vi "eMbot Testing Shift Register.vi"() -> ()   [LabVIEW 2011]
uses:
  C:/Users/mouli/Desktop/Desktop Items/Peter/Peter LabView VIs/eMbot testing/eMbot Benchtop Testing/USDQSB.dll
  USDQSB.dll
  Marker Tracking/subVIs/Global Save.vi
  <vilib>/Utility/file.llb/Write To Spreadsheet File (string).vi
panel:
  out "appended path":path
  in  "Trial":dbl=1.0
  out "Execution:State":T1(ring)
  in  "Subject ID":string="A1234"
  in  "Target Time":dbl=60.0
  out "Elspsed Time":dbl
  in  "Save Location":path=path "C:/Users/mouli/Desktop/Desktop Items/Peter/Data/eMbot Data"
  in  "Save":bool
  in  "stop":bool
  out "Matching Output":string[](array[string])
  in  "Plotcount":i32
  in  "Time offset":dbl
  out "Connected":bool
  out "Numeric":i32
  in  "Tab Control":T2(tab)
  in  "error in (no error)":errorcluster
  out "Signed Count":i32
  in  "Resolution 4":i32
  out "error out":errorcluster
  in  "Apply":bool
  in  "Quadrature Mode 4":enum16{"Clock and Direction", "X1", "X2", "X4"}(ring)
  out "Quadrature Mode":string="Clock and Direction"
  out "Counter Mode 4":string="Free Running"
  out "Resolution":i32=1024
  in  "Reset Count":bool caption="Reset"
  in  "Counter Mode":T3(ring)
  out "Index Configuration 4":string="Disabled"
  in  "Index Configuration":T4(ring)
  out "Trigger On Rollover":bool
  in  "OFF 8":bool caption="ON"
  out "Trigger On Rollunder":bool
  out "Trigger On Match":bool
  in  "OFF 9":bool caption="ON"
  in  "OFF 10":bool caption="ON"
  out "Trigger On Index":bool
  in  "OFF 11":bool caption="ON"
  in  "Clear Status":bool caption="Clear"
  out "Unsigned Count":u32
  out "Status (hex)":u32 format="%x"
  out "Rollover":bool
  out "Rollunder":bool
  out "Match":bool
  out "Index":bool
  out "Counter Enabled":bool
  out "Count Increase":bool
  out "Sign Bit Set":bool
  out "Enable Counter":bool=TRUE
  in  "OFF 12":bool=TRUE caption="ON"
  out "Invert Direction":bool=TRUE
  in  "OFF":bool=TRUE caption="ON"
  out "Encoder Count":dbl(knob) scale=0.0..1023.0
  in  "Connect":bool
  out "Connection Status":string
  in  "Port Name i.e. COM3":string="COM4"
  out "ConnectOpened":bool
  out "ConnectOpened 2":bool
  in  "Port Name i.e. COM3 2":string="COM5"
  out "error out 2":errorcluster
  in  "error in (no error) 2":errorcluster
  in  "Reset Count 2":bool caption="Reset"
  out "Encoder Count 2":dbl(knob) scale=0.0..1023.0
  in  "Clear Status 2":bool caption="Clear"
  out "Unsigned Count 2":u32
  out "Sign Bit Set 2":bool
  out "Count Increase 2":bool
  out "Counter Enabled   2":bool
  out "Index 2":bool
  out "Match 2":bool
  out "Rollunder 2":bool
  out "Rollover 2":bool
  out "Status (hex)    2":u32 format="%x"
  out "Invert Direction 2":bool
  out "Enable Counter 2":bool
  out "Trigger On Index 2":bool
  out "Trigger On Match 2":bool
  out "Trigger On Rollunder 2":bool
  out "Trigger On Rollover 2":bool
  out "Index Configuration 2":string="Disabled"
  out "Counter Mode 2":string="Free Running"
  out "Quadrature Mode 2":string="Clock and Direction"
  out "Resolution 2":i32=1024
  in  "Apply 2":bool caption="Apply"
  in  "OFF 2":bool caption="ON"
  in  "OFF 3":bool=TRUE caption="ON"
  in  "OFF 4":bool caption="ON"
  in  "OFF 5":bool caption="ON"
  in  "OFF 6":bool caption="ON"
  in  "OFF 7":bool caption="ON"
  in  "Index Configuration 3":T4(ring)
  in  "Counter Mode 3":T3(ring)
  in  "Quadrature Mode 3":enum16{"Clock and Direction", "X1", "X2", "X4"}(ring)
  out "Signed Count 2":i32
  in  "Resolution 3":i32
  in  "Have Save\nToggle Begin":bool
  in  "Phase":dbl(slide) scale=0.0..180.0
  in  "Amplitude":dbl(slide)=50.0 scale=0.0..180.0
  in  "Frequency":dbl(slide)=5.0 min=0.0 max=10.0 step=0.01 scale=0.0..10.0
  in  "Offset":dbl(slide)=50.0 scale=0.0..180.0
  in  "Slave Arm":bool
  out "Gait 2":cluster{i32, dbl}[](graph)
  out "Plot":cluster{"Gait 2":cluster{i32, dbl}[]}[](graph)
  in  "Begin":bool
  in  "EMG?":bool
  in  "Popup":bool
  in  "Publish":bool
  in  "Notes":string
  # "COM4: Rainbow cord\nCOM5: Purple cord"
  # "Encoder Configuration"
  # "Encoder Status"
  # "Encoder Configuration"
  # "COM 4"
  # "COM 5"
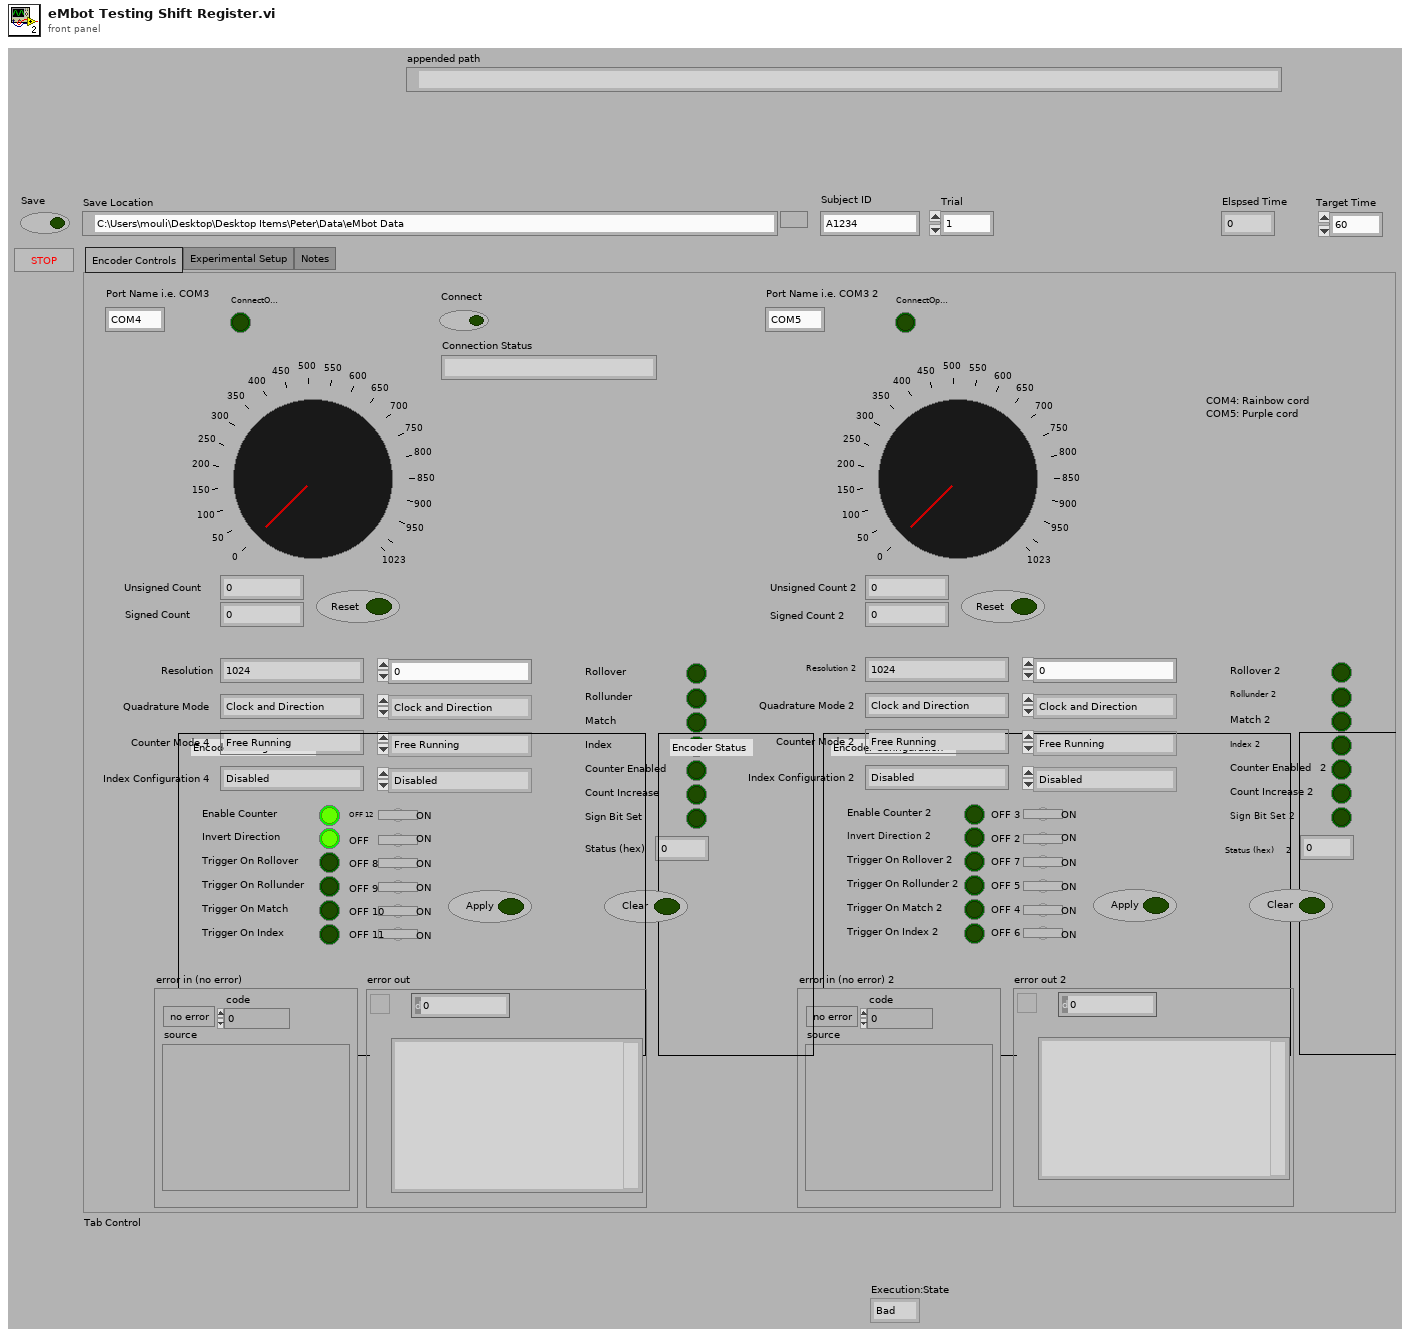
[diagram p1: front panel]
types:
  T1 = enum32{"Bad", "Idle", "Run top level", "Running"}
  T2 = enum32{"Encoder Controls", "Experimental Setup", "Notes"}
  T3 = enum16{"Free Running", "Non-Recycle", "Range Limit", "Modulo-N"}
  T4 = enum16{"Disabled", "Preset Counter", "Reset Counter", "Capture Counter"}
  T5 = enum32{"Invalid", "Standard", "Closed", "Hidden", "Minimized", "Maximized"}
  T6 = typedef "LVDateTimeRec.ctl" = cluster{"fractional second":dbl, "second":i32, "minute":i32, "hour":i32, "day of month":i32, "month":i32, "year":i32, "day of week":i32, "day of year":i32, "DST":i32}
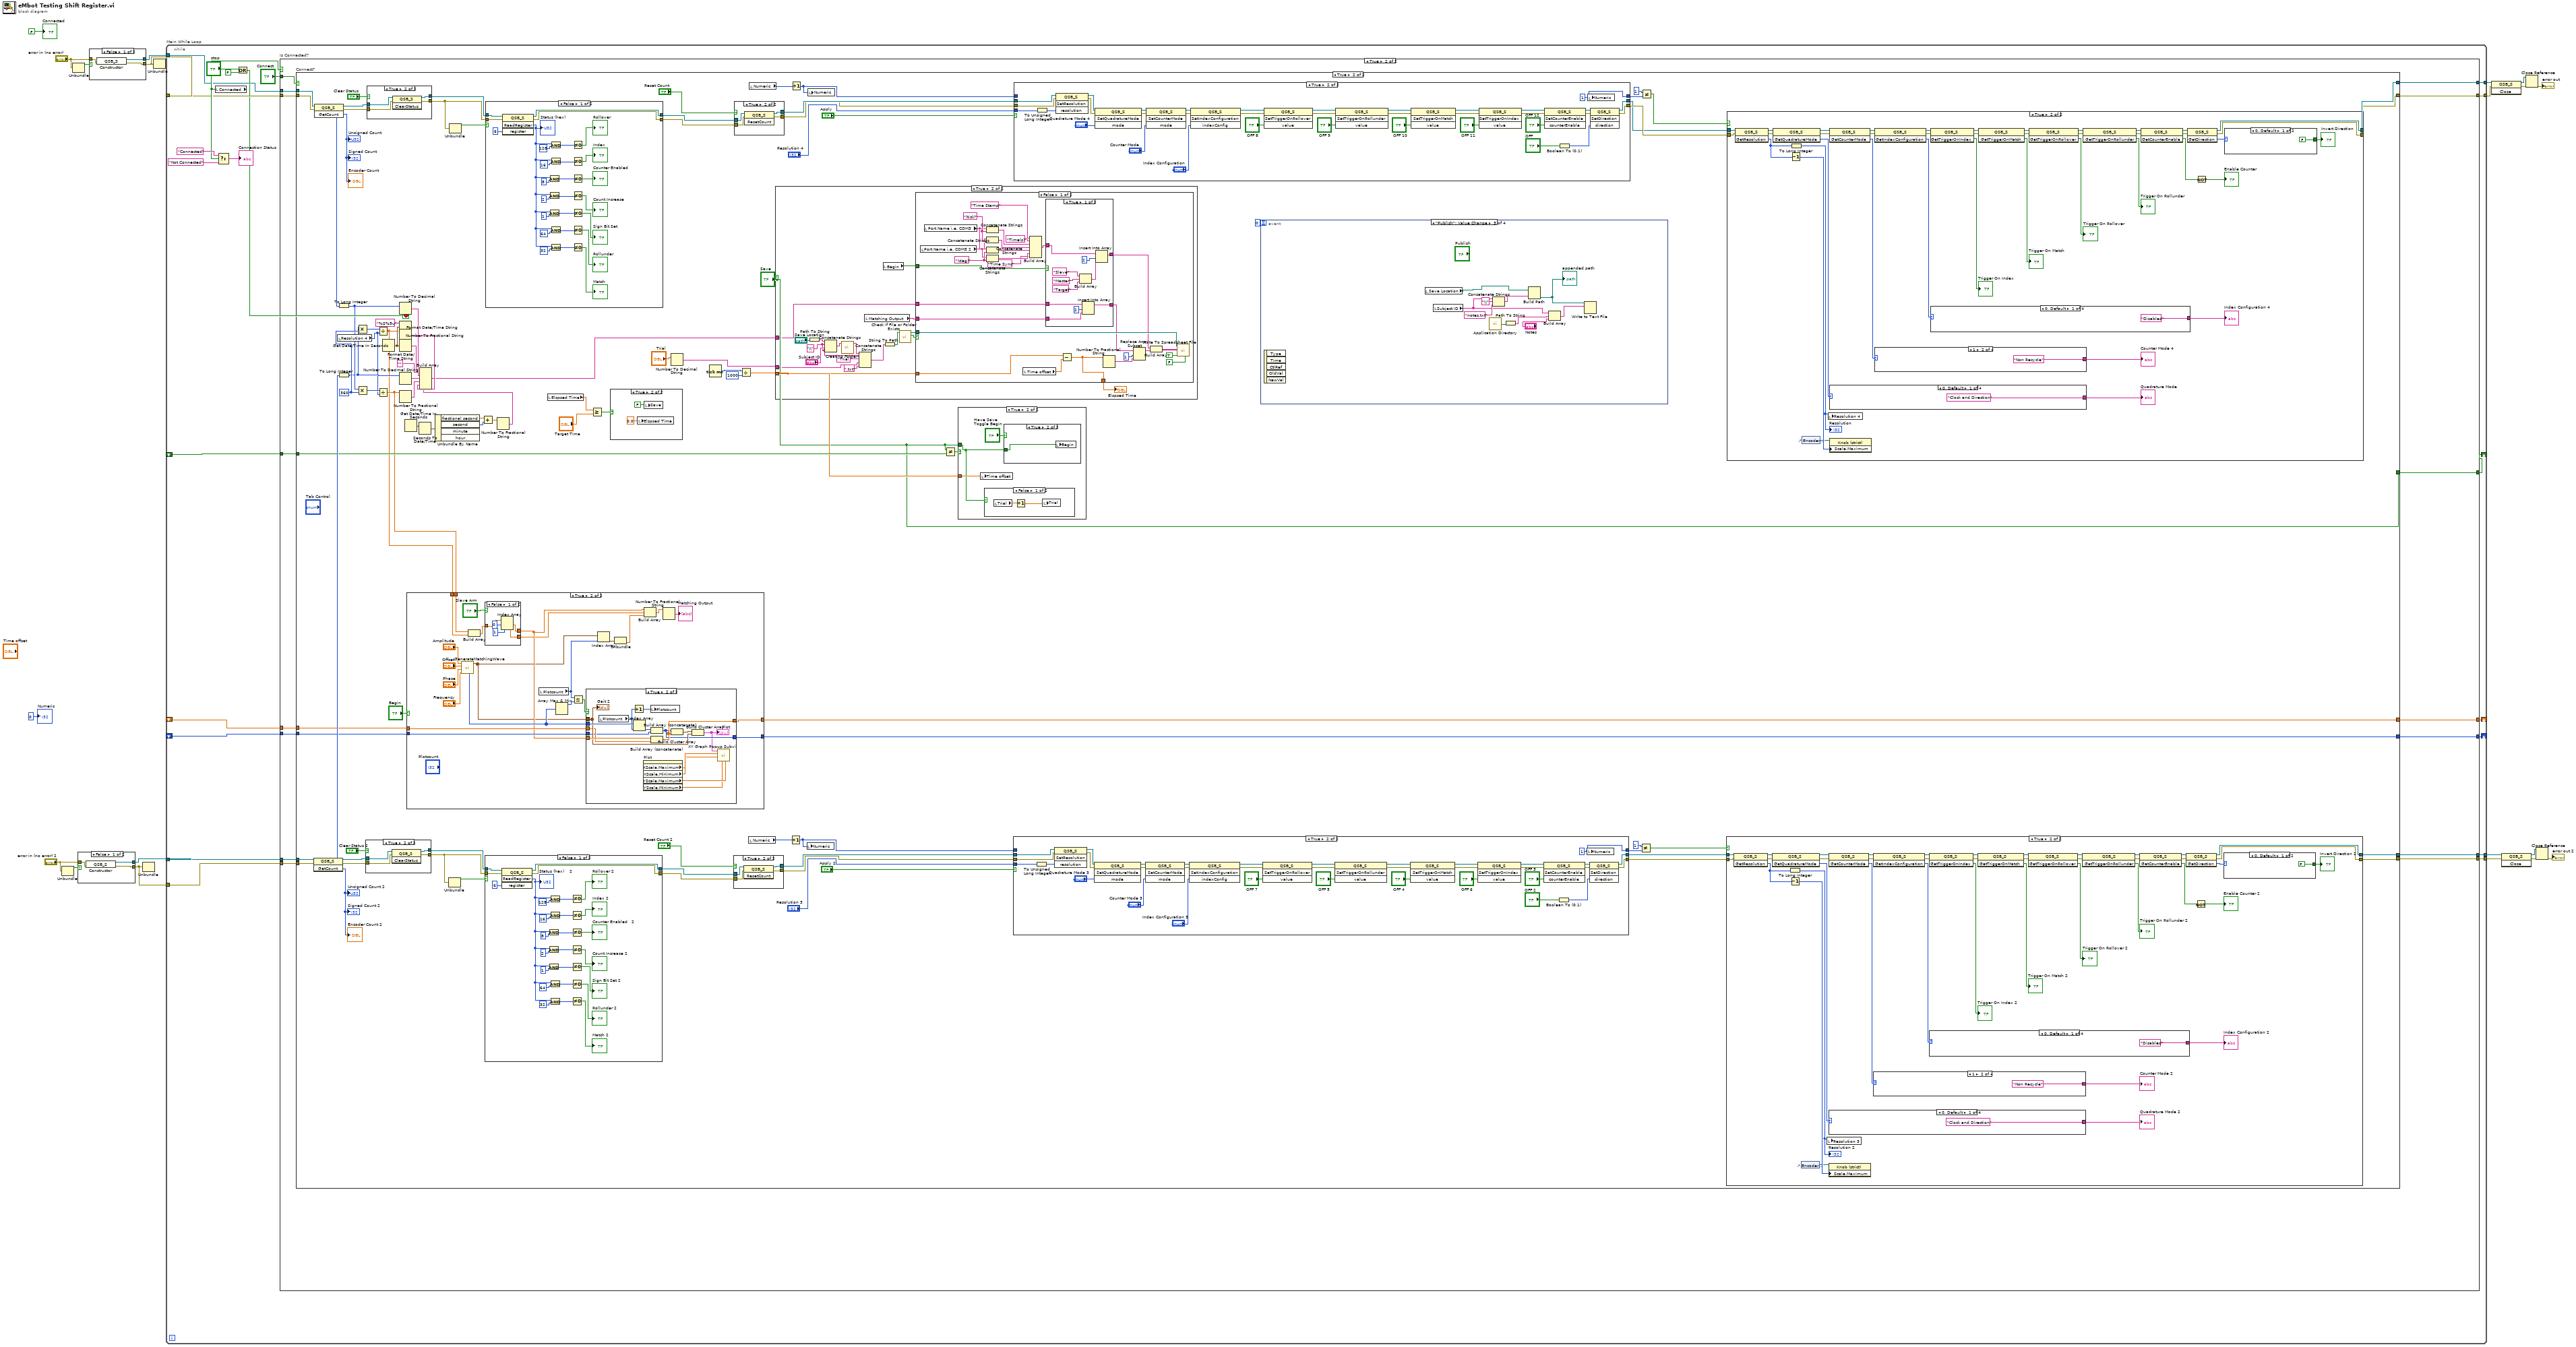
[diagram p0: block diagram]
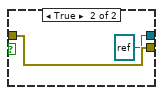
[diagram p2: hidden frame]
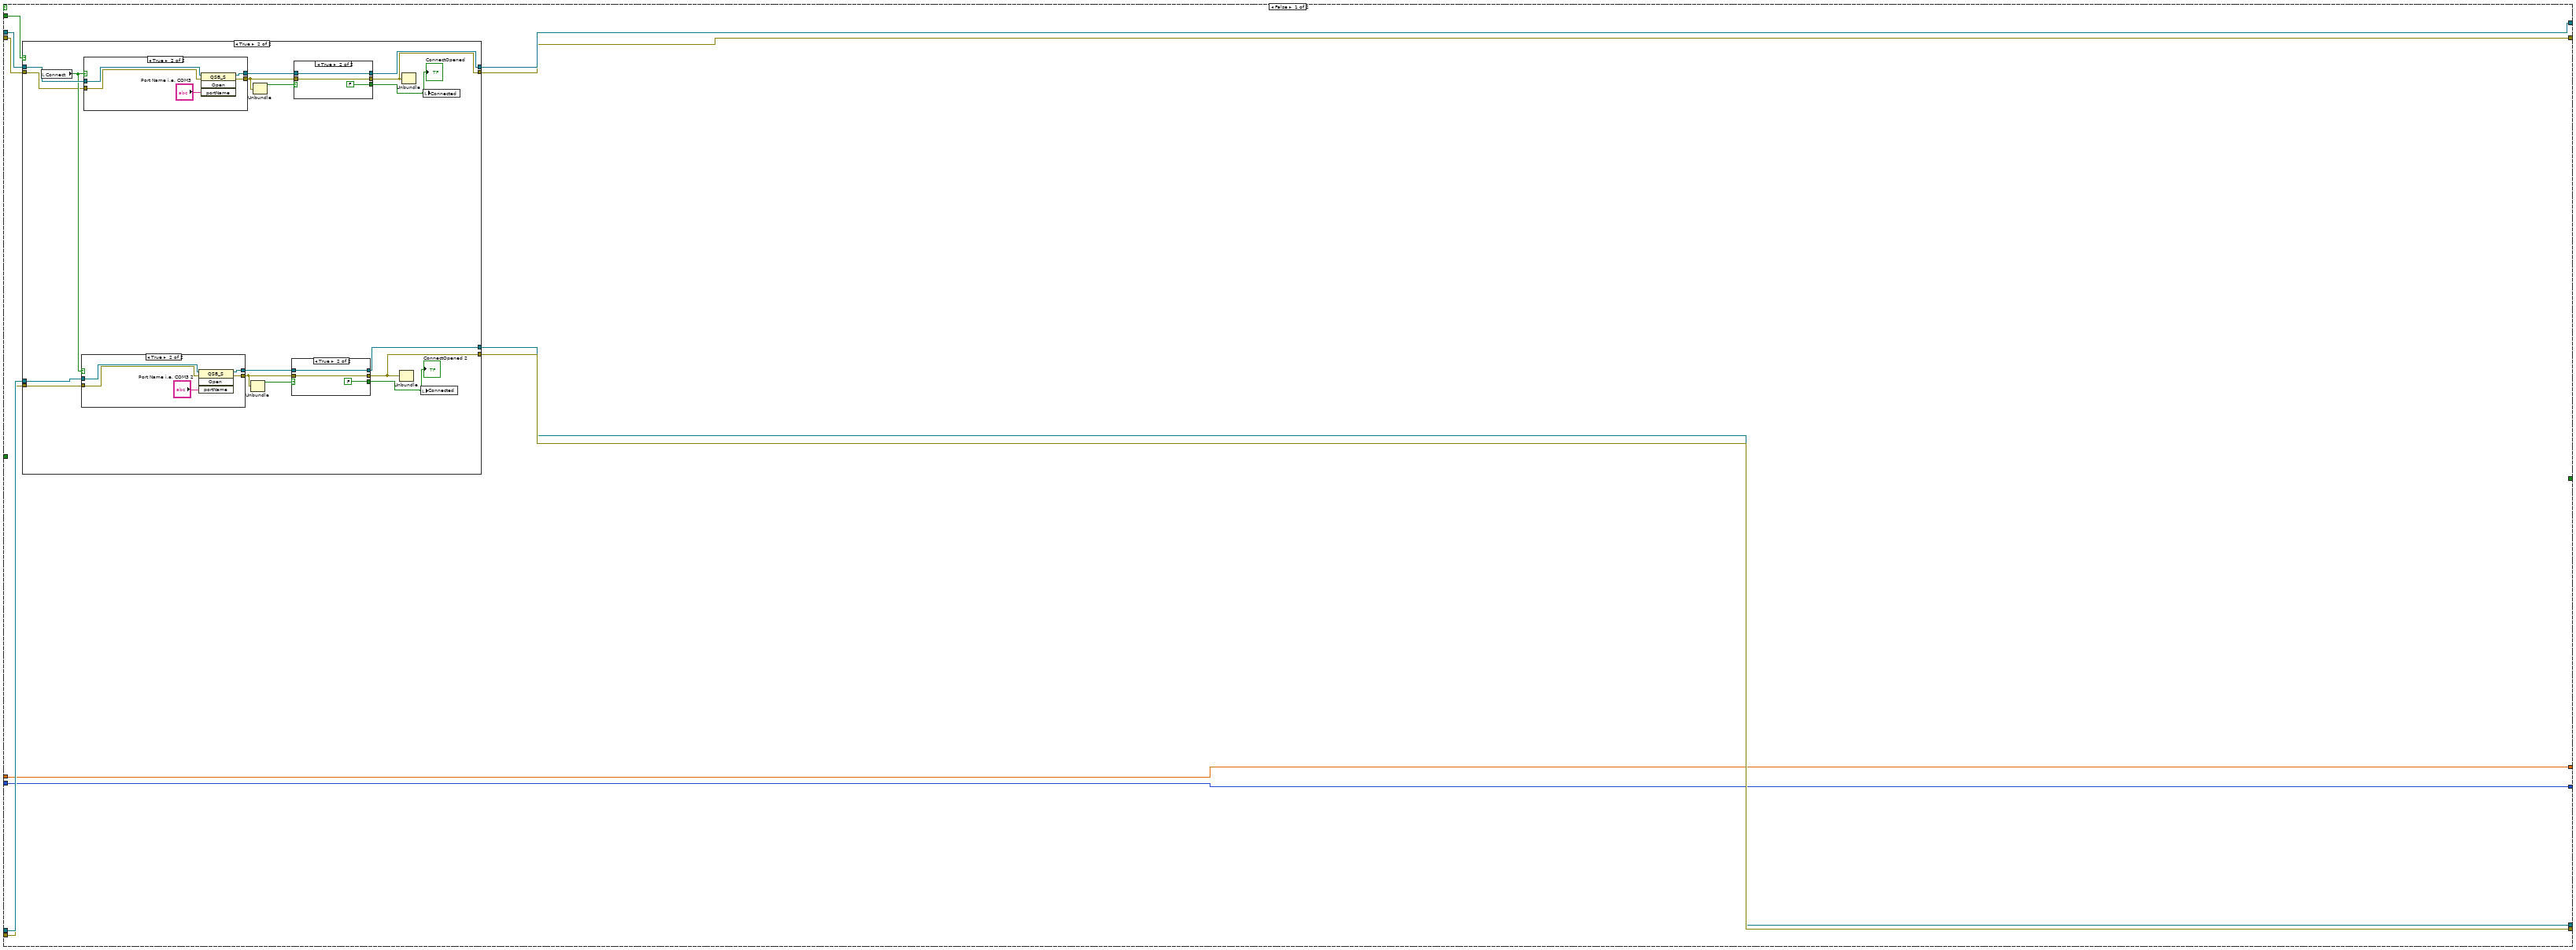
[diagram p3: hidden frame]
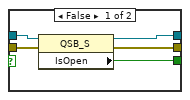
[diagram p5: hidden frame]
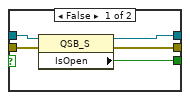
[diagram p7: hidden frame]
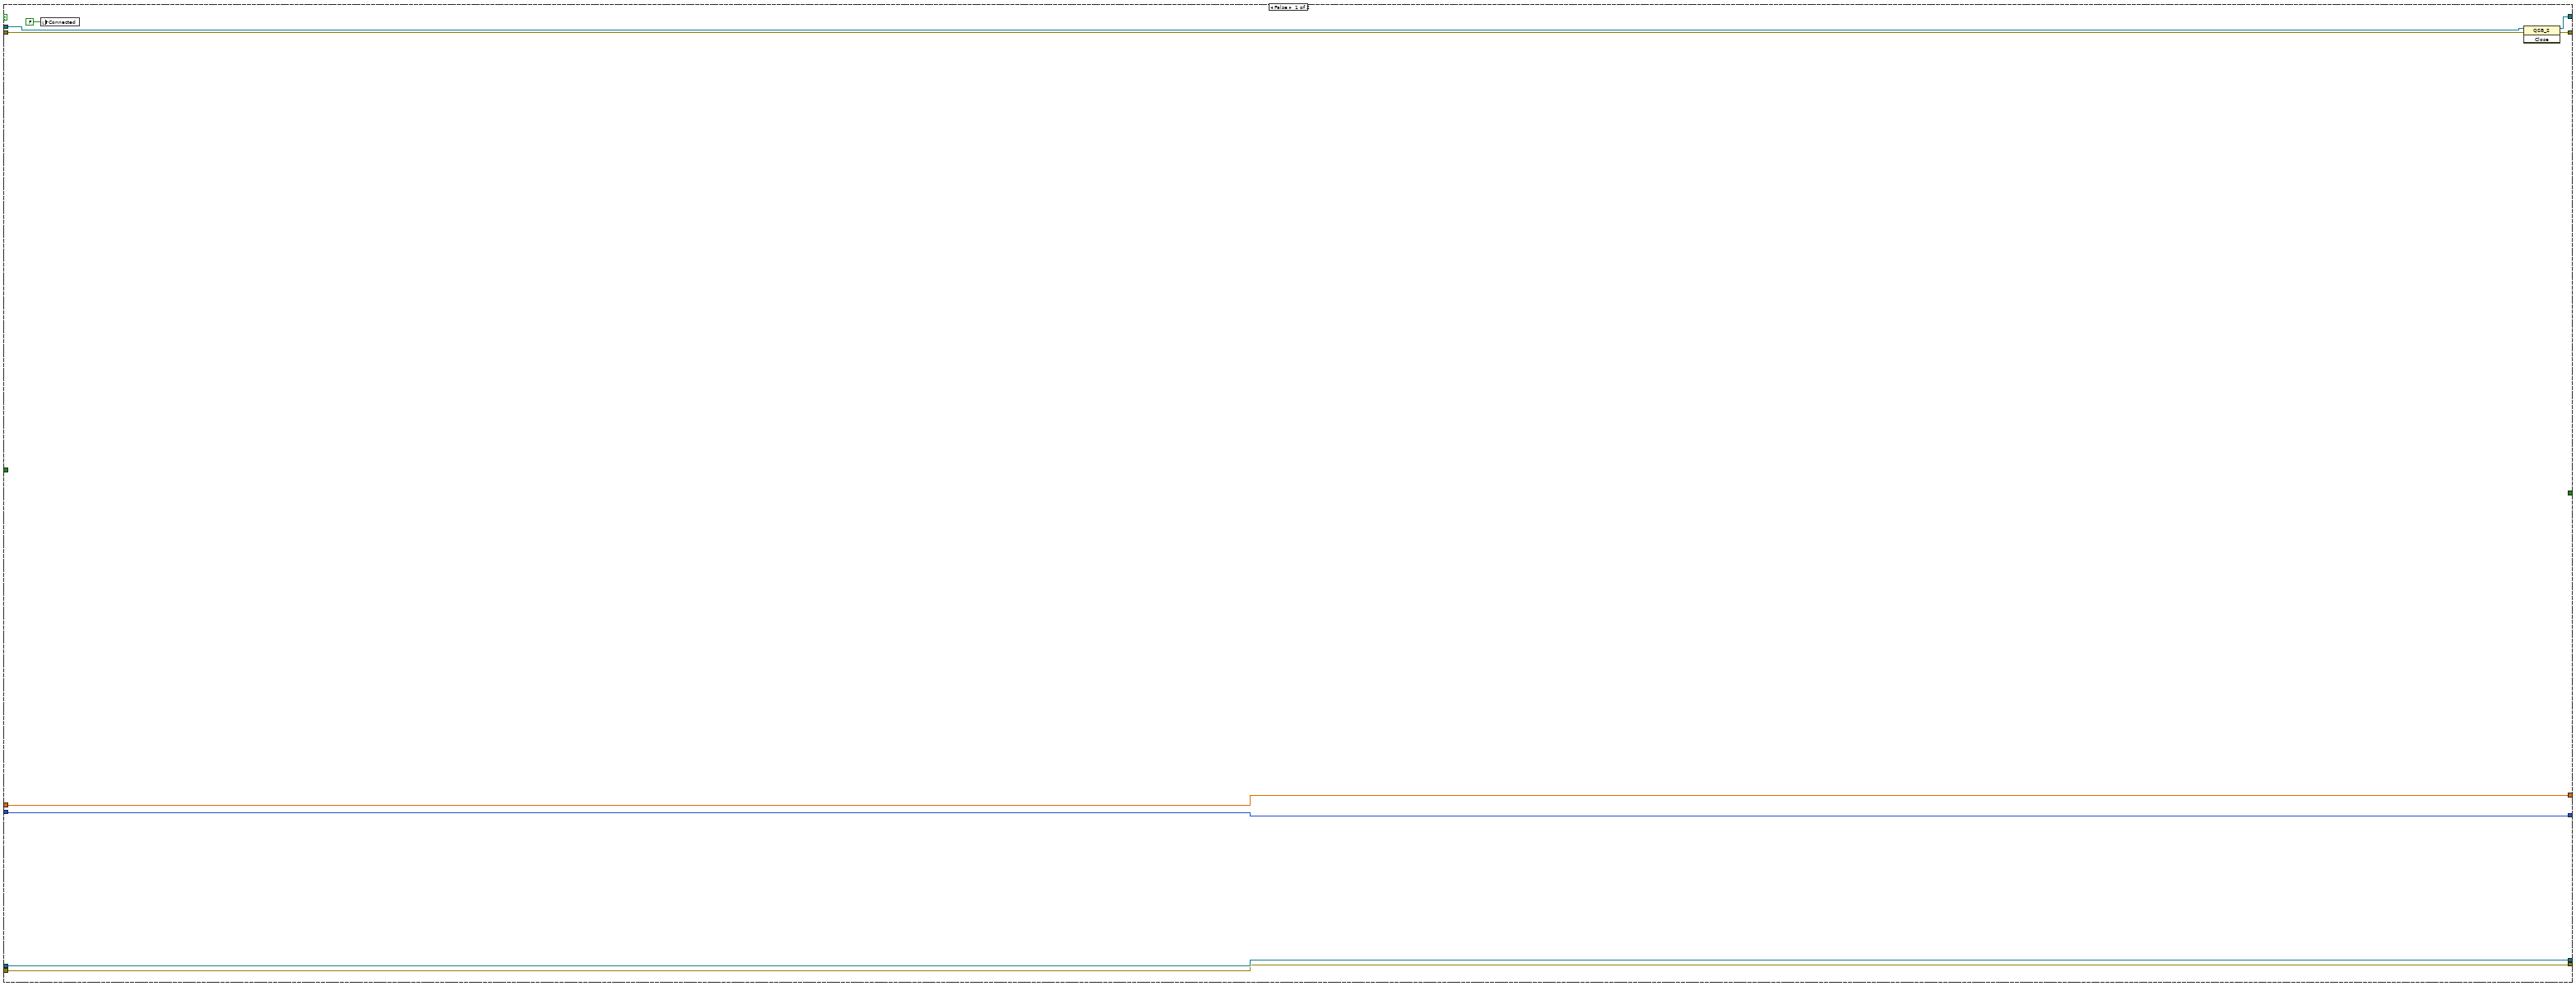
[diagram p9: hidden frame]
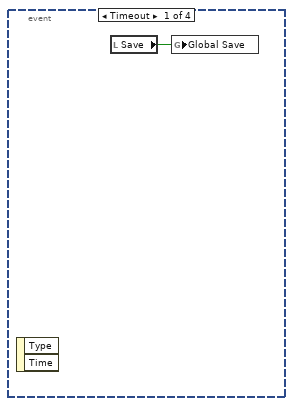
[diagram p10: hidden frame]
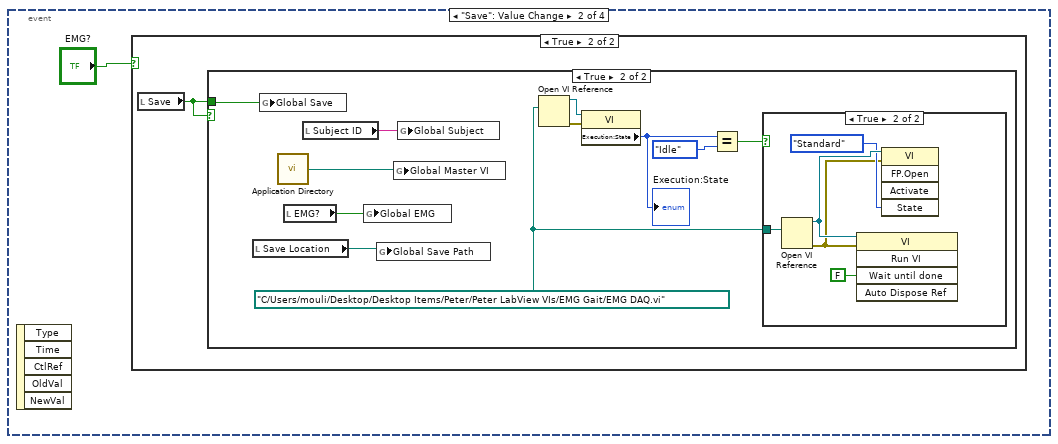
[diagram p11: hidden frame]
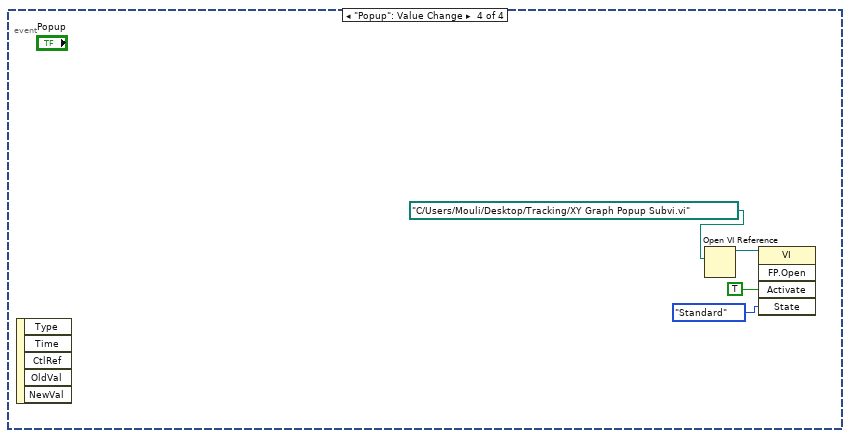
[diagram p15: hidden frame]
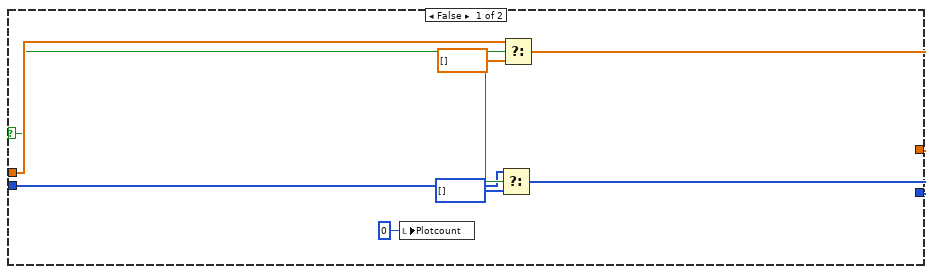
[diagram p17: hidden frame]
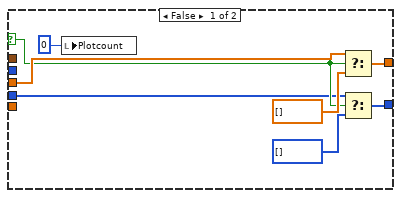
[diagram p18: hidden frame]
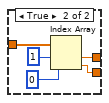
[diagram p19: hidden frame]
diagram:
  n1 = Unbundle("error in (no error) 2") -> ("status"=w3:bool)  [unwired: 2 out]
  n2 = Unbundle("error in (no error)") -> ("status"=w20:bool)  [unwired: 2 out]
  n3 = case shown="False" w3 {
    tunnel: [w21 refnum<k24> refnum ("new reference")] -> w2
    tunnel: "error in (no error) 2" -> [w23 w25]
    tunnel: [w22 w25] -> w1
    frame False {
      n4 = constructor class="QSB_S"(error in=w23) -> (reference out=w21:refnum<k24>, error out=w22:errorcluster)  [unwired: 2 in, 1 out]
    }
    frame True {
    }
  }
  n5 = case shown="False" w20 {
    tunnel: [w26 refnum<k24> refnum ("new reference")] -> w12
    tunnel: "error in (no error)" -> [w28 w30]
    tunnel: [w27 w30] -> w11
    frame False {
      n6 = constructor class="QSB_S"(error in=w28) -> (reference out=w26:refnum<k24>, error out=w27:errorcluster)  [unwired: 2 in, 1 out]
    }
    frame True {
    }
  }
  n7 = Unbundle(w1) -> ()  [unwired: 3 out]
  n8 = Unbundle(w11) -> ()  [unwired: 3 out]
  n9 = while "Main While Loop" {
    tunnel: [w52] -> w15
    tunnel: [w51] -> w14
    tunnel: w12 -> [w45]
    tunnel: w11 -> [w44]
    tunnel: [w40] -> w6
    tunnel: [w39] -> w5
    tunnel: w2 -> [w38]
    tunnel: w1 -> [w37]
    shift-right: [w36] -> _
    shift-left: _ -> [w35]
    shift-right: [w33] -> _
    shift-left: _ -> [w34]
    shift-right: [w31] -> _
    shift-left: _ -> [w32]
    stop <- w43 stop-if-true
    n10 = local read "Connected"() -> (w48:bool)
    n11 = Select(t="Connected", s=w48, f="Not Connected") -> (s? t:f=→"Connection Status":string)
    n12 = Or(x="stop", y=FALSE) -> (x .or. y?=w43:bool)
    n13 = case "Is Connected?" shown="True" w48 {
      tunnel: [w60 w127] -> w52
      tunnel: [w59 w126] -> w51
      tunnel: "Connect" -> [w63 w125]
      tunnel: w45 -> [w62 w123]
      tunnel: w44 -> [w61 w124]
      tunnel: [w58 w119] -> w40
      tunnel: [w57 w120] -> w39
      tunnel: w38 -> [w56 w122]
      tunnel: w37 -> [w55 w121]
      tunnel: [_ w118] -> w36
      tunnel: w35 -> [_ w117]
      tunnel: w34 -> [w54 w116]
      tunnel: [w54 w115] -> w33
      tunnel: w32 -> [w53 w114]
      tunnel: [w53 w113] -> w31
      frame False {
        n14 = case shown="True" w63 {
          tunnel: w62 -> [w64 w72]
          tunnel: w61 -> [w65 w70]
          tunnel: [w65 w77] -> w59
          tunnel: [w64 w78] -> w60
          tunnel: [w64 w69] -> w57
          tunnel: [w65 w68] -> w58
          tunnel: w56 -> [_ w67]
          tunnel: w55 -> [_ w66]
          frame False {
          }
          frame True {
            n15 = local read "Connect"() -> (w71:bool)
            n16 = case shown="True" w71 {
              tunnel: [w92 w97] -> w74
              tunnel: [w91 w96] -> w75
              tunnel: w67 -> [w92 w94]
              tunnel: w66 -> [w91 w93]
              frame False {
              }
              frame True {
                n17 = invoke class="QSB_S" method="Open"(reference=w94, error in=w93, "portName"="Port Name i.e. COM3 2") -> (reference out=w97:refnum<k24>, error out=w96:errorcluster)  [unwired: 1 in, 2 out]
              }
            }
            n18 = case shown="True" w71 {
              tunnel: [w107 w112] -> w81
              tunnel: [w106 w111] -> w80
              tunnel: w72 -> [w107 w109]
              tunnel: w70 -> [w106 w108]
              frame False {
              }
              frame True {
                n19 = invoke class="QSB_S" method="Open"(reference=w109, error in=w108, "portName"="Port Name i.e. COM3") -> (reference out=w112:refnum<k24>, error out=w111:errorcluster)  [unwired: 1 in, 2 out]
              }
            }
            n20 = Unbundle(w75) -> ("status"=w73:bool)  [unwired: 2 out]
            n21 = Unbundle(w80) -> ("status"=w82:bool)  [unwired: 2 out]
            n22 = case shown="True" w73 {
              tunnel: [w87 w89] -> w69
              tunnel: [w86 w90] -> w68
              tunnel: w74 -> [w84 w89]
              tunnel: w75 -> [w85 w90]
              tunnel: [w83 FALSE] -> w76
              frame False {
                n23 = property class="QSB_S"(reference=w84, error in=w85) -> (reference out=w87:refnum<k24>, error out=w86:errorcluster, "IsOpen"=w83:bool)
              }
              frame True {
              }
            }
            "ConnectOpened 2" <- w76
            n24 = case shown="True" w82 {
              tunnel: [w102 w104] -> w78
              tunnel: [w101 w105] -> w77
              tunnel: w81 -> [w99 w104]
              tunnel: w80 -> [w100 w105]
              tunnel: [w98 FALSE] -> w79
              frame False {
                n25 = property class="QSB_S"(reference=w99, error in=w100) -> (reference out=w102:refnum<k24>, error out=w101:errorcluster, "IsOpen"=w98:bool)
              }
              frame True {
              }
            }
            "ConnectOpened" <- w79
            n26 = Unbundle(w68) -> ()  [unwired: 3 out]
            n27 = Unbundle(w77) -> ()  [unwired: 3 out]
            n28 = local write "Connected"(w76) -> ()
            n29 = local write "Connected"(w79) -> ()
          }
        }
      }
      frame True {
        n30 = case "Connect?" shown="True" w125 {
          tunnel: [w133 w223] -> w127
          tunnel: [w134 w222] -> w126
          tunnel: w124 -> [w136 w211]
          tunnel: w123 -> [w135 w210]
          tunnel: w122 -> [w131 w182]
          tunnel: w121 -> [w130 w181]
          tunnel: [w131 w180] -> w120
          tunnel: [w130 w179] -> w119
          tunnel: [_ "Save"] -> w118
          tunnel: w117 -> [_ w160]
          tunnel: w116 -> [w129 w154]
          tunnel: [w129 w153] -> w115
          tunnel: w114 -> [w128 w152]
          tunnel: [w128 w151] -> w113
          frame False {
            n31 = local write "Connected"(FALSE) -> ()
            n32 = invoke class="QSB_S" method="Close"(reference=w135, error in=w136) -> (reference out=w133:refnum<k24>, error out=w134:errorcluster)  [unwired: 1 in, 1 out]
          }
          frame True {
            w172 = 360 ("y")
            n33 = invoke class="QSB_S" method="GetCount"(reference=w182, error in=w181) -> (reference out=w197:refnum<k24>, error out=w196:errorcluster, "GetCount"=w165:u32)  [unwired: 1 in]
            "Signed Count 2" <- w165
            "Unsigned Count 2" <- w165
            "Encoder Count 2" <- w165
            n34 = invoke class="QSB_S" method="GetCount"(reference=w210, error in=w211) -> (reference out=w208:refnum<k24>, error out=w209:errorcluster, "GetCount"=w167:u32)  [unwired: 1 in]
            "Signed Count" <- w167
            "Unsigned Count" <- w167
            "Encoder Count" <- w167
            n35 = local read "Resolution 4"() -> (w163:i32)
            n36 = To Long Integer(number=w167) -> (32bit integer=w166:i32)
            n37 = To Long Integer(number=w165) -> (32bit integer=w164:i32)
            n38 = Multiply(x=w164, y=w172) -> (x*y=w176:i32)
            n39 = Multiply(x=w166, y=w172) -> (x*y=w174:i32)
            n40 = case shown="True" "Clear Status 2" {
              tunnel: [w415 w419] -> w190
              tunnel: [w416 w417] -> w191
              tunnel: w197 -> [w415 w420]
              tunnel: w196 -> [w416 w418]
              frame False {
              }
              frame True {
                n41 = invoke class="QSB_S" method="ClearStatus"(reference=w420, error in=w418) -> (reference out=w419:refnum<k24>, error out=w417:errorcluster)  [unwired: 1 in, 1 out]
              }
            }
            n42 = case shown="True" "Clear Status" {
              tunnel: [w550 w554] -> w217
              tunnel: [w551 w552] -> w216
              tunnel: w208 -> [w550 w555]
              tunnel: w209 -> [w551 w553]
              frame False {
              }
              frame True {
                n43 = invoke class="QSB_S" method="ClearStatus"(reference=w555, error in=w553) -> (reference out=w554:refnum<k24>, error out=w552:errorcluster)  [unwired: 1 in, 1 out]
              }
            }
            n44 = Divide(x=w176, y=w163) -> (x/y=w157:dbl)
            n45 = Divide(x=w174, y=w163) -> (x/y=w158:dbl)
            n46 = Get Date/Time In Seconds() -> (seconds since 1Jan1904=w170:timestamp)
            n47 = Number To Decimal String(number=w166) -> (decimal integer string=w178:string)  [unwired: 1 in]
            n48 = Format Date/Time String(time format string (%c)="%S%5u", seconds (now)=w170) -> ()  [unwired: 1 in, 1 out]
            n49 = Number To Fractional String(number=w157) -> (F-format string=w175:string)  [unwired: 3 in]
            n50 = Format Date/Time String(seconds (now)=w170) -> (date/time string=w169:string)  [unwired: 2 in]
            n51 = Number To Decimal String(number=w164) -> (decimal integer string=w177:string)  [unwired: 1 in]
            n52 = Number To Fractional String(number=w158) -> (F-format string=w173:string)  [unwired: 3 in]
            n53 = Get Date/Time In Seconds() -> (seconds since 1Jan1904=w144:timestamp)
            n54 = case shown="True" "Begin" {
              selector: "Begin" -> [w267 _]
              tunnel: w158 -> [_ w292]
              tunnel: w157 -> [_ w291]
              tunnel: w154 -> [w268 w281]
              tunnel: [w262 w280] -> w153
              tunnel: w152 -> [w266 w279]
              tunnel: [w263 w278] -> w151
              frame False {
                n55 = local write "Plotcount"(0 ("Plotcount")) -> ()
                n56 = Select(t=w266, s=w267, f=i32[] []) -> (s? t:f=w263:i32[])
                n57 = Select(t=w268, s=w267, f=dbl[] []) -> (s? t:f=w262:dbl[])
              }
              frame True {
                n58 = call "GenerateMatchingWave.vi"("Frequency"="Frequency", "phase in"="Phase", "Offset"="Offset", "Amplitude"="Amplitude") -> ("Gait 2"=w274:cluster{i32, dbl}[], "X Scale"=w282:i32[])  [unwired: 6 in]
                n59 = Build Array(w292, w291) -> (w290:dbl[])
                n60 = case shown="False" "Slave Arm" {
                  tunnel: w290 -> [w321 w326]
                  tunnel: [w319 w324] -> w277
                  tunnel: [w317 w322] -> w276
                  frame False {
                    n61 = Index Array(array=w321, index #1=0 ("index"), index #2=1 ("index")) -> (element #1=w319:dbl, element #2=w317:dbl)
                  }
                  frame True {
                    n62 = Index Array(array=w326, index #1=1 ("index"), index #2=0 ("index")) -> (element #1=w324:dbl, element #2=w322:dbl)
                  }
                }
                n63 = local read "Plotcount"() -> (w273:i32)
                n64 = Array Max & Min(array=w282) -> (max value=w283:i32)  [unwired: 3 out]
                n65 = Less Or Equal?(x=w273, y=w283) -> (x <= y?=w284:bool)
                n66 = case shown="True" w284 {
                  selector: w284 -> [w296 _]
                  tunnel: w277 -> [_ w316]
                  tunnel: w274 -> [_ w310]
                  tunnel: w282 -> [_ w313]
                  tunnel: w281 -> [w299 w309]
                  tunnel: [w297 w308] -> w280
                  tunnel: w279 -> [w295 w307]
                  tunnel: [w293 w306] -> w278
                  frame False {
                    n67 = local write "Plotcount"(0 ("Plotcount")) -> ()
                    n68 = Select(t=w299, s=w296, f=dbl[] []) -> (s? t:f=w297:dbl[])
                    n69 = Select(t=w295, s=w296, f=i32[] []) -> (s? t:f=w293:i32[])
                  }
                  frame True {
                    n70 = local read "Plotcount"() -> (w312:i32)
                    n71 = Increment(x=w312) -> (x+1=w314:i32)
                    n72 = Index Array(array=w313, index=w312) -> (element=w311:i32)
                    n73 = property on="Plot" class="XYGraph (strict)"() -> ("XScale.Maximum"=w303:dbl, "XScale.Minimum"=w304:dbl, "YScale.Maximum"=w302:dbl, "YScale.Minimum"=w301:dbl)  [unwired: 2 in, 2 out]
                    n74 = local write "Plotcount"(w314) -> ()
                    n75 = Build Array (concatenate)(w311, w307) -> (w306:i32[])
                    n76 = Build Array (concatenate)(w316, w309) -> (w308:dbl[])
                    n77 = Build Cluster Array(w306, w308) -> (w315:cluster{i32, dbl}[])
                    n78 = Build Cluster Array(w315, w310) -> (w305:cluster{"Gait 2":cluster{i32, dbl}[]}[])
                    "Plot" <- w305
                    n79 = call "XY Graph Popup Subvi.vi"("Y Scale.Range:Maximum"=w302, "Y Scale.Range:Minimum"=w301, "X Scale.Range:Maximum"=w303, "X Scale.Range:Minimum"=w304, 11:w305) -> ()  [unwired: 6 in, 1 out]
                    "Gait 2" <- w310
                  }
                }
                n80 = Index Array(array=w274, index=w273) -> (element=w272:cluster{i32, dbl})
                n81 = Unbundle(w272) -> (w271:dbl)  [unwired: 1 out]
                n82 = Build Array(w277, w276, w271) -> (w275:dbl[])
                n83 = Number To Fractional String(number=w275) -> (F-format string=→"Matching Output":string[])  [unwired: 3 in]
              }
            }
            n84 = Seconds To Date/Time(time stamp (now)=w144) -> (date time rec=w143:T6)  [unwired: 1 in]
            n85 = Unbundle By Name(w143) -> ("fractional second"=w142:dbl, "second"=w141:i32)  [unwired: 2 out]
            n86 = Unbundle(w191) -> ("status"=w188:bool)  [unwired: 2 out]
            n87 = Unbundle(w216) -> ("status"=w219:bool)  [unwired: 2 out]
            n88 = Add(x=w142, y=w141) -> (x+y=w140:dbl)
            n89 = case shown="False" w188 {
              tunnel: w191 -> [w447 w449]
              tunnel: w190 -> [w446 w448]
              tunnel: [w445 w448] -> w199
              tunnel: [w443 w449] -> w198
              frame False {
                n90 = invoke on="Invoke Node" class="QSB_S" method="ReadRegister"(reference=w446, error in=w447, "register"=6) -> (reference out=w445:refnum<k24>, error out=w443:errorcluster, "ReadRegister"=w421:u32)  [unwired: 1 in, 1 out]
                "Status (hex)    2" <- w421
                n91 = And(x=w421, y=8) -> (x .and. y?=w429:u32)
                n92 = And(x=w421, y=2) -> (x .and. y?=w426:u32)
                n93 = And(x=w421, y=1) -> (x .and. y?=w423:u32)
                n94 = And(x=w421, y=128) -> (x .and. y?=w441:u32)
                n95 = And(x=w421, y=16) -> (x .and. y?=w432:u32)
                n96 = And(x=w421, y=64) -> (x .and. y?=w438:u32)
                n97 = And(x=w421, y=32) -> (x .and. y?=w435:u32)
                n98 = Not Equal To 0?(x=w441) -> (x != 0?=→"Rollover 2":bool)
                n99 = Not Equal To 0?(x=w432) -> (x != 0?=→"Index 2":bool)
                n100 = Not Equal To 0?(x=w429) -> (x != 0?=→"Counter Enabled   2":bool)
                n101 = Not Equal To 0?(x=w426) -> (x != 0?=→"Count Increase 2":bool)
                n102 = Not Equal To 0?(x=w423) -> (x != 0?=→"Sign Bit Set 2":bool)
                n103 = Not Equal To 0?(x=w438) -> (x != 0?=→"Rollunder 2":bool)
                n104 = Not Equal To 0?(x=w435) -> (x != 0?=→"Match 2":bool)
              }
              frame True {
              }
            }
            n105 = case shown="False" w219 {
              tunnel: w216 -> [w582 w584]
              tunnel: w217 -> [w581 w583]
              tunnel: [w580 w583] -> w206
              tunnel: [w578 w584] -> w207
              frame False {
                n106 = invoke on="Invoke Node" class="QSB_S" method="ReadRegister"(reference=w581, error in=w582, "register"=6) -> (reference out=w580:refnum<k24>, error out=w578:errorcluster, "ReadRegister"=w556:u32)  [unwired: 1 in, 1 out]
                "Status (hex)" <- w556
                n107 = And(x=w556, y=8) -> (x .and. y?=w564:u32)
                n108 = And(x=w556, y=2) -> (x .and. y?=w561:u32)
                n109 = And(x=w556, y=1) -> (x .and. y?=w558:u32)
                n110 = And(x=w556, y=128) -> (x .and. y?=w576:u32)
                n111 = And(x=w556, y=16) -> (x .and. y?=w567:u32)
                n112 = And(x=w556, y=64) -> (x .and. y?=w573:u32)
                n113 = And(x=w556, y=32) -> (x .and. y?=w570:u32)
                n114 = Not Equal To 0?(x=w576) -> (x != 0?=→"Rollover":bool)
                n115 = Not Equal To 0?(x=w567) -> (x != 0?=→"Index":bool)
                n116 = Not Equal To 0?(x=w564) -> (x != 0?=→"Counter Enabled":bool)
                n117 = Not Equal To 0?(x=w561) -> (x != 0?=→"Count Increase":bool)
                n118 = Not Equal To 0?(x=w558) -> (x != 0?=→"Sign Bit Set":bool)
                n119 = Not Equal To 0?(x=w573) -> (x != 0?=→"Rollunder":bool)
                n120 = Not Equal To 0?(x=w570) -> (x != 0?=→"Match":bool)
              }
              frame True {
              }
            }
            n121 = Number To Fractional String(number=w140) -> (F-format string=w139:string)  [unwired: 3 in]
            n122 = Build Array(w169, "" ("element"), w178, w177, w173, w175, w139) -> (w150:string[])
            n123 = local read "Elspsed Time"() -> (w149:dbl)
            n124 = Greater Or Equal?(x=w149, y="Target Time") -> (x >= y?=w147:bool)
            n125 = case shown="True" w147 {
              frame False {
              }
              frame True {
                n126 = local write "Elspsed Time"(0.0 ("Elspsed Time")) -> ()
                n127 = local write "Save"(FALSE ("Save")) -> ()
              }
            }
            n128 = Number To Decimal String(number="Trial") -> (decimal integer string=w137:string)  [unwired: 1 in]
            n129 = Tick Count (ms)() -> (millisecond timer value=w162:u32)
            n130 = case shown="True" "Reset Count 2" {
              tunnel: w198 -> [w409 w414]
              tunnel: w199 -> [w410 w413]
              tunnel: [w410 w412] -> w200
              tunnel: [w409 w411] -> w201
              frame False {
              }
              frame True {
                n131 = invoke class="QSB_S" method="ResetCount"(reference=w413, error in=w414) -> (reference out=w412:refnum<k24>, error out=w411:errorcluster)  [unwired: 1 in, 1 out]
              }
            }
            n132 = case shown="True" "Reset Count" {
              tunnel: w207 -> [w544 w549]
              tunnel: w206 -> [w545 w548]
              tunnel: [w545 w547] -> w205
              tunnel: [w544 w546] -> w204
              frame False {
              }
              frame True {
                n133 = invoke class="QSB_S" method="ResetCount"(reference=w548, error in=w549) -> (reference out=w547:refnum<k24>, error out=w546:errorcluster)  [unwired: 1 in, 1 out]
              }
            }
            n134 = Divide(x=w162, y=u32 1000) -> (x/y=w156:dbl)
            n135 = local read "Numeric"() -> (w186:i32)
            n136 = local read "Numeric"() -> (w221:i32)
            n137 = case shown="True" "Save" {
              tunnel: w150 -> [_ w350]
              tunnel: w156 -> [_ w346]
              tunnel: w137 -> [_ w337]
              frame False {
              }
              frame True {
                w338 = "\\" ("string")
                n138 = Path To String(path="Save Location") -> (string=w333:string)
                n139 = Concatenate Strings(w333, w338, "Subject ID", w338) -> (w341:string)
                n140 = call "Creating Folder.vi"("Input String Path"=w341) -> ("Output String Path"=w335:string)  [unwired: 10 in]
                n141 = Concatenate Strings(w335, w338, "Trial " ("string"), w337, ".txt" ("string")) -> (w340:string)
                n142 = local read "Matching Output"() -> (w344:string[])
                n143 = local read "Begin"() -> (w345:bool)
                n144 = String To Path(string=w340) -> (path=w349:path)
                n145 = call <vilib>:"Check if File or Folder Exists.vi"("path"=w349) -> ("file or folder exists?"=w348:bool, "dup path"=w347:path)  [unwired: 8 in, 1 out]
                n146 = case shown="False" w348 {
                  tunnel: w347 -> [w377 w402]
                  tunnel: w350 -> [w367 w393]
                  tunnel: w346 -> [w369 w400]
                  tunnel: w345 -> [w365 w395]
                  tunnel: w344 -> [w364 w394]
                  tunnel: [w352 w391] -> w343
                  frame False {
                    w357 = "(deg)"
                    w360 = "(tick)"
                    n147 = local read "Port Name i.e. COM3 2"() -> (w356:string)
                    n148 = local read "Port Name i.e. COM3"() -> (w358:string)
                    n149 = Concatenate Strings(w358, w360) -> (w361:string)
                    n150 = Concatenate Strings(w356, w360) -> (w359:string)
                    n151 = Concatenate Strings(w358, w357) -> (w354:string)
                    n152 = Concatenate Strings(w356, w357) -> (w355:string)
                    n153 = local read "Time offset"() -> (w368:dbl)
                    n154 = Build Array("Time Stamp", "Time(s)", w361, w359, w354, w355, "Time Sync" ("element")) -> (w353:string[])
                    n155 = case shown="True" w365 {
                      tunnel: [w384 w389] -> w375
                      tunnel: w367 -> [w383 w390]
                      tunnel: [w381 w390] -> w366
                      tunnel: w364 -> [w380 _]
                      tunnel: w353 -> [w378 w389]
                      frame True {
                        n156 = Build Array("Slave", "Master", "Target") -> (w386:string[])
                        n157 = Insert Into Array(array=w383, index=2, new element=w380) -> (w381:string[])
                        n158 = Insert Into Array(array=w378, index=2, new element=w386) -> (w384:string[])
                      }
                      frame False {
                      }
                    }
                    n159 = Subtract(x=w369, y=w368) -> (x-y=w352:dbl)
                    n160 = Number To Fractional String(number=w352) -> (F-format string=w372:string)  [unwired: 3 in]
                    n161 = Replace Array Subset(array=w366, new element=w372, index=1) -> (w370:string[])
                    n162 = Build Array(w375, w370) -> (w374:string[][])
                    n163 = call-poly <vilib>:"Write To Spreadsheet File.vi"("transpose? (no:F)"=FALSE, "append to file? (new file:F)"=TRUE, "2D data"=w374, "file path (dialog if empty)"=w377) -> ()  [unwired: 4 in, 1 out]
                  }
                  frame True {
                    n164 = case shown="False" w395 {
                      tunnel: w394 -> [_ w406]
                      tunnel: w393 -> [w404 w408]
                      tunnel: [w404 w405] -> w392
                      frame False {
                      }
                      frame True {
                        n165 = Insert Into Array(array=w408, index=2, new element=w406) -> (w405:string[])
                      }
                    }
                    n166 = local read "Time offset"() -> (w399:dbl)
                    n167 = Subtract(x=w400, y=w399) -> (x-y=w391:dbl)
                    n168 = Number To Fractional String(number=w391) -> (F-format string=w397:string)  [unwired: 3 in]
                    n169 = Replace Array Subset(array=w392, new element=w397, index=1) -> (w396:string[])
                    n170 = call-poly <vilib>:"Write To Spreadsheet File.vi"("transpose? (no:F)"=FALSE, "append to file? (new file:F)"=TRUE, "1D data"=w396, "file path (dialog if empty)"=w402) -> ()  [unwired: 4 in, 1 out]
                  }
                }
                "Elspsed Time" <- w343
              }
            }
            n171 = Increment(x=w186) -> (x+1=w187:i32)
            n172 = Increment(x=w221) -> (x+1=w220:i32)
            n173 = local write "Numeric"(w187) -> ()
            n174 = local write "Numeric"(w220) -> ()
            n175 = Not Equal?(x="Save", y=w160) -> (x != y?=w159:bool)
            n176 = case shown="True" w159 {
              tunnel: w156 -> [_ w329]
              tunnel: "Save" -> [_ w327]
              frame False {
              }
              frame True {
                n177 = local write "Time offset"(w329) -> ()
                n178 = case shown="False" w327 {
                  frame False {
                    n179 = local read "Trial"() -> (w331:dbl)
                    n180 = Increment(x=w331) -> (x+1=w330:dbl)
                    n181 = local write "Trial"(w330) -> ()
                  }
                  frame True {
                  }
                }
                n182 = case shown="True" "Have Save\nToggle Begin" {
                  tunnel: w327 -> [_ w332]
                  frame False {
                  }
                  frame True {
                    n183 = local write "Begin"(w332) -> ()
                  }
                }
              }
            }
            n184 = case shown="True" "Apply 2" {
              tunnel: w201 -> [w508 w543]
              tunnel: w200 -> [w507 w542]
              tunnel: [w507 w510] -> w185
              tunnel: [w508 w509] -> w184
              tunnel: "Resolution 3" -> [_ w541]
              tunnel: w187 -> [w506 _]
              tunnel: [w506 w534] -> w194
              frame False {
              }
              frame True {
                w534 = 1
                n185 = To Unsigned Long Integer(number=w541) -> (unsigned 32bit integer=w511:u32)
                n186 = invoke class="QSB_S" method="SetResolution"(reference=w542, error in=w543, "resolution"=w511) -> (reference out=w540:refnum<k24>, error out=w539:errorcluster)  [unwired: 1 in, 2 out]
                n187 = invoke class="QSB_S" method="SetQuadratureMode"(reference=w540, error in=w539, "mode"="Quadrature Mode 3") -> (reference out=w538:refnum<k24>, error out=w537:errorcluster)  [unwired: 1 in, 2 out]
                n188 = invoke class="QSB_S" method="SetCounterMode"(reference=w538, error in=w537, "mode"="Counter Mode 3") -> (reference out=w536:refnum<k24>, error out=w535:errorcluster)  [unwired: 1 in, 2 out]
                n189 = invoke class="QSB_S" method="SetIndexConfiguration"(reference=w536, error in=w535, "indexConfig"="Index Configuration 3") -> (reference out=w530:refnum<k24>, error out=w529:errorcluster)  [unwired: 1 in, 2 out]
                n190 = invoke class="QSB_S" method="SetTriggerOnRollover"(reference=w530, error in=w529, "value"="OFF 7") -> (reference out=w533:refnum<k24>, error out=w528:errorcluster)  [unwired: 1 in, 2 out]
                n191 = invoke class="QSB_S" method="SetTriggerOnRollunder"(reference=w533, error in=w528, "value"="OFF 5") -> (reference out=w532:refnum<k24>, error out=w527:errorcluster)  [unwired: 1 in, 2 out]
                n192 = invoke class="QSB_S" method="SetTriggerOnMatch"(reference=w532, error in=w527, "value"="OFF 4") -> (reference out=w531:refnum<k24>, error out=w526:errorcluster)  [unwired: 1 in, 2 out]
                n193 = invoke class="QSB_S" method="SetTriggerOnIndex"(reference=w531, error in=w526, "value"="OFF 6") -> (reference out=w515:refnum<k24>, error out=w512:errorcluster)  [unwired: 1 in, 2 out]
                n194 = invoke class="QSB_S" method="SetCounterEnable"(reference=w515, error in=w512, "counterEnable"="OFF 3") -> (reference out=w514:refnum<k24>, error out=w513:errorcluster)  [unwired: 1 in, 2 out]
                n195 = Boolean To (0,1)(Boolean="OFF 2") -> (0, 1=w516:i16)
                n196 = local write "Numeric"(w534) -> ()
                n197 = invoke class="QSB_S" method="SetDirection"(reference=w514, error in=w513, "direction"=w516) -> (reference out=w510:refnum<k24>, error out=w509:errorcluster)  [unwired: 1 in, 2 out]
              }
            }
            n198 = case shown="True" "Apply" {
              tunnel: w204 -> [w643 w678]
              tunnel: w205 -> [w642 w677]
              tunnel: [w642 w645] -> w224
              tunnel: [w643 w644] -> w225
              tunnel: "Resolution 4" -> [_ w676]
              tunnel: w220 -> [w641 _]
              tunnel: [w641 w669] -> w213
              frame False {
              }
              frame True {
                w669 = 1
                n199 = To Unsigned Long Integer(number=w676) -> (unsigned 32bit integer=w646:u32)
                n200 = invoke class="QSB_S" method="SetResolution"(reference=w677, error in=w678, "resolution"=w646) -> (reference out=w675:refnum<k24>, error out=w674:errorcluster)  [unwired: 1 in, 2 out]
                n201 = invoke class="QSB_S" method="SetQuadratureMode"(reference=w675, error in=w674, "mode"="Quadrature Mode 4") -> (reference out=w673:refnum<k24>, error out=w672:errorcluster)  [unwired: 1 in, 2 out]
                n202 = invoke class="QSB_S" method="SetCounterMode"(reference=w673, error in=w672, "mode"="Counter Mode") -> (reference out=w671:refnum<k24>, error out=w670:errorcluster)  [unwired: 1 in, 2 out]
                n203 = invoke class="QSB_S" method="SetIndexConfiguration"(reference=w671, error in=w670, "indexConfig"="Index Configuration") -> (reference out=w665:refnum<k24>, error out=w664:errorcluster)  [unwired: 1 in, 2 out]
                n204 = invoke class="QSB_S" method="SetTriggerOnRollover"(reference=w665, error in=w664, "value"="OFF 8") -> (reference out=w668:refnum<k24>, error out=w663:errorcluster)  [unwired: 1 in, 2 out]
                n205 = invoke class="QSB_S" method="SetTriggerOnRollunder"(reference=w668, error in=w663, "value"="OFF 9") -> (reference out=w667:refnum<k24>, error out=w662:errorcluster)  [unwired: 1 in, 2 out]
                n206 = invoke class="QSB_S" method="SetTriggerOnMatch"(reference=w667, error in=w662, "value"="OFF 10") -> (reference out=w666:refnum<k24>, error out=w661:errorcluster)  [unwired: 1 in, 2 out]
                n207 = invoke class="QSB_S" method="SetTriggerOnIndex"(reference=w666, error in=w661, "value"="OFF 11") -> (reference out=w650:refnum<k24>, error out=w647:errorcluster)  [unwired: 1 in, 2 out]
                n208 = invoke class="QSB_S" method="SetCounterEnable"(reference=w650, error in=w647, "counterEnable"="OFF 12") -> (reference out=w649:refnum<k24>, error out=w648:errorcluster)  [unwired: 1 in, 2 out]
                n209 = Boolean To (0,1)(Boolean="OFF") -> (0, 1=w651:i16)
                n210 = local write "Numeric"(w669) -> ()
                n211 = invoke class="QSB_S" method="SetDirection"(reference=w649, error in=w648, "direction"=w651) -> (reference out=w645:refnum<k24>, error out=w644:errorcluster)  [unwired: 1 in, 2 out]
              }
            }
            n212 = event shown="[2] \"Publish\": Value Change" {
              selector: _ -> [_ _ _ _]
              dyn-events: _ -> [_ _ _ _]
              timeout: 0 -> [_ _ _ _]
              event Timeout {
                n213 = event-data() -> ()  [unwired: 1 in, 2 out]
                n214 = local read "Save"() -> (w227:bool)
                n215 = global write "Global Save.vi" "Global Save"(w227) -> ()
              }
              event "Save": Value Change {
                n216 = event-data() -> ()  [unwired: 1 in, 5 out]
                n217 = case shown="True" "EMG?" {
                  frame False {
                  }
                  frame True {
                    n218 = local read "Save"() -> (w229:bool)
                    n219 = case shown="True" w229 {
                      tunnel: w229 -> [_ w240]
                      frame False {
                      }
                      frame True {
                        w239 = path "C:/Users/mouli/Desktop/Desktop Items/Peter/Peter LabView VIs/EMG Gait/EMG DAQ.vi" ("vi path")
                        n220 = local read "Save Location"() -> (w230:path)
                        n221 = global write "Global Save.vi" "Global Save"(w240) -> ()
                        n222 = call <vilib>:"Application Directory.vi"() -> ("Application Directory"=w232:path)
                        n223 = local read "EMG?"() -> (w231:bool)
                        n224 = local read "Subject ID"() -> (w233:string)
                        n225 = global write "Global Save.vi" "Global EMG"(w231) -> ()
                        n226 = global write "Global Save.vi" "Global Save Path"(w230) -> ()
                        n227 = global write "Global Save.vi" "Global Master VI"(w232) -> ()
                        n228 = global write "Global Save.vi" "Global Subject"(w233) -> ()
                        n229 = Open VI Reference(vi path=w239) -> (vi reference=w238:refnum<vi>, error out=w234:errorcluster)  [unwired: 5 in]
                        n230 = property class="VI"(reference=w238, error in=w234) -> ("Execution:State"=w237:T1)  [unwired: 2 out]
                        "Execution:State" <- w237
                        n231 = Equal?(x=w237, y=T1."Idle") -> (x = y?=w235:bool)
                        n232 = case shown="True" w235 {
                          tunnel: w239 -> [_ w241]
                          frame False {
                          }
                          frame True {
                            n233 = Open VI Reference(vi path=w241) -> (vi reference=w244:refnum<vi>, error out=w242:errorcluster)  [unwired: 5 in]
                            n234 = invoke class="VI" method="Run VI"(reference=w244, error in=w242, "Wait until done"=FALSE ("Activate?")) -> ()  [unwired: 2 in, 5 out]
                            n235 = invoke class="VI" method="FP.Open"(reference=w244, error in=w242, "State"=T5."Standard") -> ()  [unwired: 2 in, 5 out]
                          }
                        }
                      }
                    }
                  }
                }
              }
              event "Publish": Value Change {
                n236 = event-data() -> ()  [unwired: 1 in, 5 out]
                n237 = local read "Save Location"() -> (w246:path)
                n238 = local read "Subject ID"() -> (w249:string)
                n239 = call <vilib>:"Application Directory.vi"() -> ("Application Directory"=w253:path)
                n240 = Concatenate Strings(w249, "\\" ("string"), "notes.txt" ("name or relative path")) -> (w247:string)
                n241 = Path To String(path=w253) -> (string=w255:string)
                n242 = Build Path(base path=w246, name or relative path=w247) -> (appended path=w251:path)
                "appended path" <- w251
                n243 = Build Array(w249, w255, "Notes") -> (w252:string[])
                n244 = Write to Text File(file (use dialog)=w251, text=w252) -> ()  [unwired: 2 in, 3 out]
              }
              event "Popup": Value Change {
                n245 = event-data() -> ()  [unwired: 1 in, 5 out]
                n246 = Open VI Reference(vi path=path "C:/Users/Mouli/Desktop/Tracking/XY Graph Popup Subvi.vi") -> (vi reference=w256:refnum<vi>)  [unwired: 5 in, 1 out]
                n247 = invoke class="VI" method="FP.Open"(reference=w256, "Activate"=TRUE ("Activate?"), "State"=T5."Standard") -> ()  [unwired: 2 in, 5 out]
              }
            }
            n248 = Not Equal?(x=1, y=w194) -> (x != y?=w195:bool)
            n249 = Not Equal?(x=1, y=w213) -> (x != y?=w212:bool)
            n250 = case shown="True" w195 {
              tunnel: w184 -> [w451 w491]
              tunnel: w185 -> [w450 w490]
              tunnel: [w450 w461] -> w180
              tunnel: [w451 w460] -> w179
              frame False {
              }
              frame True {
                n251 = invoke class="QSB_S" method="GetResolution"(reference=w490, error in=w491) -> (reference out=w489:refnum<k24>, error out=w487:errorcluster, "GetResolution"=w454:u32)  [unwired: 1 in]
                n252 = invoke class="QSB_S" method="GetQuadratureMode"(reference=w489, error in=w487) -> (reference out=w488:refnum<k24>, error out=w486:errorcluster, "GetQuadratureMode"=w484:i32)  [unwired: 1 in]
                n253 = To Long Integer(number=w454) -> (32bit integer=w452:i32)
                "Resolution 2" <- w452
                n254 = Decrement(x=w454) -> (x-1=w455:u32)
                n255 = control-ref of="Encoder Count 2"() -> (w453:refnum<vi>)
                n256 = local write "Resolution 3"(w452) -> ()
                n257 = invoke class="QSB_S" method="GetCounterMode"(reference=w488, error in=w486) -> (reference out=w481:refnum<k24>, error out=w480:errorcluster, "GetCounterMode"=w483:i32)  [unwired: 1 in]
                n258 = case shown="0, Default" w484 {
                  tunnel: ["Clock and Direction" "X1" "X2" "X4"] -> w485
                  frame 0, Default {
                  }
                  frame 1 {
                  }
                  frame 2 {
                  }
                  frame 3 {
                  }
                }
                "Quadrature Mode 2" <- w485
                n259 = property on="Property Node" class="Knob (strict)"(reference=w453, "Scale.Maximum"=w455) -> ()  [unwired: 1 in, 2 out]
                n260 = invoke class="QSB_S" method="GetIndexConfiguration"(reference=w481, error in=w480) -> (reference out=w477:refnum<k24>, error out=w473:errorcluster, "GetIndexConfiguration"=w479:i32)  [unwired: 1 in]
                n261 = case shown="1" w483 {
                  tunnel: ["Free Running" "Non Recycle" "Range Limit" "Modulo-N"] -> w482
                  frame 0 {
                  }
                  frame 1 {
                  }
                  frame 2 {
                  }
                  frame 3, Default {
                  }
                }
                "Counter Mode 2" <- w482
                n262 = invoke class="QSB_S" method="GetTriggerOnIndex"(reference=w477, error in=w473) -> (reference out=w476:refnum<k24>, error out=w472:errorcluster, "GetTriggerOnIndex"=→"Trigger On Index 2":bool)  [unwired: 1 in]
                n263 = case shown="0, Default" w479 {
                  tunnel: ["Disabled" "Preset Counter" "Reset Counter" "Capture Counter"] -> w478
                  frame 0, Default {
                  }
                  frame 1 {
                  }
                  frame 2 {
                  }
                  frame 3 {
                  }
                }
                "Index Configuration 2" <- w478
                n264 = invoke class="QSB_S" method="GetTriggerOnMatch"(reference=w476, error in=w472) -> (reference out=w475:refnum<k24>, error out=w471:errorcluster, "GetTriggerOnMatch"=→"Trigger On Match 2":bool)  [unwired: 1 in]
                n265 = invoke class="QSB_S" method="GetTriggerOnRollover"(reference=w475, error in=w471) -> (reference out=w474:refnum<k24>, error out=w470:errorcluster, "GetTriggerOnRollover"=→"Trigger On Rollover 2":bool)  [unwired: 1 in]
                n266 = invoke class="QSB_S" method="GetTriggerOnRollunder"(reference=w474, error in=w470) -> (reference out=w465:refnum<k24>, error out=w464:errorcluster, "GetTriggerOnRollunder"=→"Trigger On Rollunder 2":bool)  [unwired: 1 in]
                n267 = invoke class="QSB_S" method="GetCounterEnable"(reference=w465, error in=w464) -> (reference out=w463:refnum<k24>, error out=w462:errorcluster, "GetCounterEnable"=w457:bool)  [unwired: 1 in]
                n268 = invoke class="QSB_S" method="GetDirection"(reference=w463, error in=w462) -> (reference out=w461:refnum<k24>, error out=w460:errorcluster, "GetDirection"=w459:i32)  [unwired: 1 in]
                n269 = Not(x=w457) -> (.not. x?=→"Enable Counter 2":bool)
                n270 = case shown="0, Default" w459 {
                  tunnel: [FALSE TRUE] -> w458
                  frame 0, Default {
                  }
                  frame 1 {
                    (unwired) "Preset Counter"
                  }
                }
                "Invert Direction 2" <- w458
              }
            }
            n271 = case shown="True" w212 {
              tunnel: w225 -> [w586 w626]
              tunnel: w224 -> [w585 w625]
              tunnel: [w585 w596] -> w223
              tunnel: [w586 w595] -> w222
              frame False {
              }
              frame True {
                n272 = invoke class="QSB_S" method="GetResolution"(reference=w625, error in=w626) -> (reference out=w624:refnum<k24>, error out=w622:errorcluster, "GetResolution"=w589:u32)  [unwired: 1 in]
                n273 = invoke class="QSB_S" method="GetQuadratureMode"(reference=w624, error in=w622) -> (reference out=w623:refnum<k24>, error out=w621:errorcluster, "GetQuadratureMode"=w619:i32)  [unwired: 1 in]
                n274 = To Long Integer(number=w589) -> (32bit integer=w587:i32)
                "Resolution" <- w587
                n275 = Decrement(x=w589) -> (x-1=w590:u32)
                n276 = control-ref of="Encoder Count"() -> (w588:refnum<vi>)
                n277 = local write "Resolution 4"(w587) -> ()
                n278 = invoke class="QSB_S" method="GetCounterMode"(reference=w623, error in=w621) -> (reference out=w616:refnum<k24>, error out=w615:errorcluster, "GetCounterMode"=w618:i32)  [unwired: 1 in]
                n279 = case shown="0, Default" w619 {
                  tunnel: ["Clock and Direction" "X1" "X2" "X4"] -> w620
                  frame 0, Default {
                  }
                  frame 1 {
                  }
                  frame 2 {
                  }
                  frame 3 {
                  }
                }
                "Quadrature Mode" <- w620
                n280 = property on="Property Node" class="Knob (strict)"(reference=w588, "Scale.Maximum"=w590) -> ()  [unwired: 1 in, 2 out]
                n281 = invoke class="QSB_S" method="GetIndexConfiguration"(reference=w616, error in=w615) -> (reference out=w612:refnum<k24>, error out=w608:errorcluster, "GetIndexConfiguration"=w614:i32)  [unwired: 1 in]
                n282 = case shown="1" w618 {
                  tunnel: ["Free Running" "Non Recycle" "Range Limit" "Modulo-N"] -> w617
                  frame 0 {
                  }
                  frame 1 {
                  }
                  frame 2 {
                  }
                  frame 3, Default {
                  }
                }
                "Counter Mode 4" <- w617
                n283 = invoke class="QSB_S" method="GetTriggerOnIndex"(reference=w612, error in=w608) -> (reference out=w611:refnum<k24>, error out=w607:errorcluster, "GetTriggerOnIndex"=→"Trigger On Index":bool)  [unwired: 1 in]
                n284 = case shown="0, Default" w614 {
                  tunnel: ["Disabled" "Preset Counter" "Reset Counter" "Capture Counter"] -> w613
                  frame 0, Default {
                  }
                  frame 1 {
                  }
                  frame 2 {
                  }
                  frame 3 {
                  }
                }
                "Index Configuration 4" <- w613
                n285 = invoke class="QSB_S" method="GetTriggerOnMatch"(reference=w611, error in=w607) -> (reference out=w610:refnum<k24>, error out=w606:errorcluster, "GetTriggerOnMatch"=→"Trigger On Match":bool)  [unwired: 1 in]
                n286 = invoke class="QSB_S" method="GetTriggerOnRollover"(reference=w610, error in=w606) -> (reference out=w609:refnum<k24>, error out=w605:errorcluster, "GetTriggerOnRollover"=→"Trigger On Rollover":bool)  [unwired: 1 in]
                n287 = invoke class="QSB_S" method="GetTriggerOnRollunder"(reference=w609, error in=w605) -> (reference out=w600:refnum<k24>, error out=w599:errorcluster, "GetTriggerOnRollunder"=→"Trigger On Rollunder":bool)  [unwired: 1 in]
                n288 = invoke class="QSB_S" method="GetCounterEnable"(reference=w600, error in=w599) -> (reference out=w598:refnum<k24>, error out=w597:errorcluster, "GetCounterEnable"=w592:bool)  [unwired: 1 in]
                n289 = invoke class="QSB_S" method="GetDirection"(reference=w598, error in=w597) -> (reference out=w596:refnum<k24>, error out=w595:errorcluster, "GetDirection"=w594:i32)  [unwired: 1 in]
                n290 = Not(x=w592) -> (.not. x?=→"Enable Counter":bool)
                n291 = case shown="0, Default" w594 {
                  tunnel: [FALSE TRUE] -> w593
                  frame 0, Default {
                  }
                  frame 1 {
                    (unwired) "Preset Counter"
                  }
                }
                "Invert Direction" <- w593
              }
            }
          }
        }
      }
    }
  }
  n292 = invoke class="QSB_S" method="Close"(reference=w15, error in=w14) -> (reference out=w17:refnum<k24>, error out=w18:errorcluster)  [unwired: 1 in, 1 out]
  n293 = invoke class="QSB_S" method="Close"(reference=w5, error in=w6) -> (reference out=w8:refnum<k24>, error out=w7:errorcluster)  [unwired: 1 in, 1 out]
  n294 = Close Reference(reference=w17, error in (no error)=w18) -> (error out=→"error out":errorcluster)
  n295 = Close Reference(reference=w8, error in (no error)=w7) -> (error out=→"error out 2":errorcluster)
  "Numeric" <- 0
  "Connected" <- FALSE
